vi "Set Transmit Start Time.vi"(10 "Tx start time":u32 format="%d us", 11 "Framework Performance in":refnum<class "Framework Performance.lvclass">) -> (3 "Framework Performance out":refnum<class "Framework Performance.lvclass">)   [LabVIEW 2017, in "Data Sharing Framework Engine.lvlib" / "Framework Performance.lvclass"]
uses:
  Framework Performance.lvclass
  Framework Performance.lvclass/Framework Performance.ctl
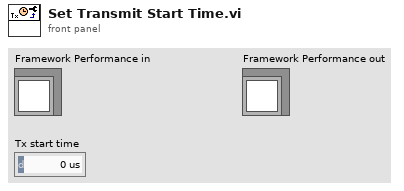
[diagram p1: front panel]
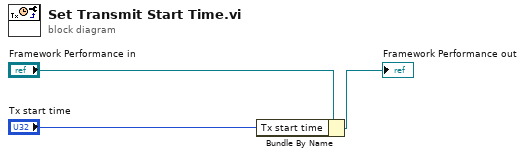
[diagram p0: block diagram]
diagram:
  n1 = Bundle By Name(cluster="Framework Performance in", "Tx start time"="Tx start time") -> (→"Framework Performance out":refnum<class "Framework Performance.lvclass">)
